vi "Configure Analog Out.vi"(0 "VISA resource name":refnum<visa-resource-name>, 1 "High Value (0.0000)":dbl min=-100000.0 max=100000.0 step=0.0001 format="%.4f", 2 "Low Value (0.0000)":dbl min=-100000.0 max=100000.0 step=0.0001 format="%.4f", 5 "Analog Out Mode (0: Off)":u16(ring) items=["Off", "Input", "Manual", "Loop 2"], 7 "Input (0: A)":u16(ring) items=["A", "B"], 9 "Source (0: Kelvin)":u16(ring) items=["Kelvin", "Celsius", "Sensor Units", "Linear Data"], 11 "error in (no error)":errorcluster, 12 "Bipolar Mode (F: OFF)":bool, 13 "Manual Value (0.000 %)":dbl min=-100.0 max=100.0 step=0.001 format="%.3f") -> (4 "VISA resource name out":refnum<visa-resource-name>, 15 "error out":errorcluster)   [LabVIEW 2013, in "Lake Shore Cryotronics 331.lvlib"]
doc: "This VI configures the 331 analog output. The analog output may be configured to send a voltage proportional to temperature to a strip chart recorder or data acquisition system The output can also be manually controlled as a voltage source for any other application or used as the countrol output for Loop 2."
uses:
  Lake Shore Cryotronics 331.lvlib
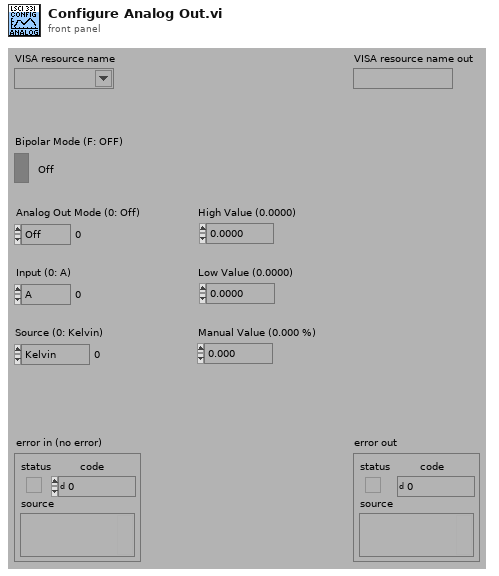
[diagram p1: front panel]
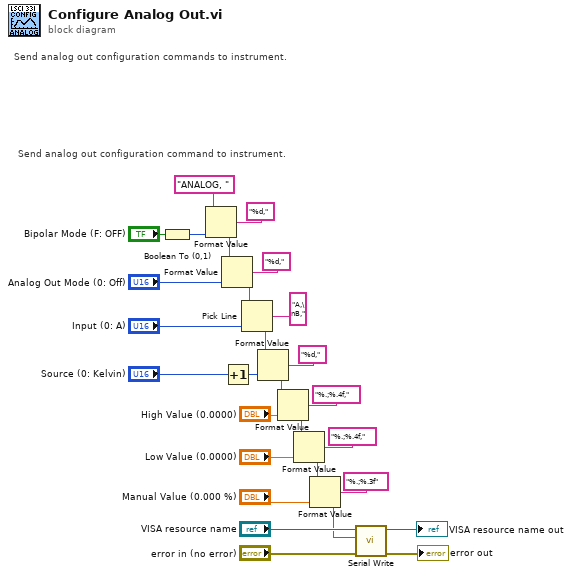
[diagram p0: block diagram]
diagram:
  # "Send analog out configuration command to instrument."
  # "Send analog out configuration commands to instrument."
  n1 = Boolean To (0,1)(Boolean="Bipolar Mode (F: OFF)") -> (0, 1=w21:i16)
  n2 = Format Value(string ("")="ANALOG, ", format string="%d,", value (0)=w21) -> (output string=w18:string)
  n3 = Format Value(string ("")=w18, format string="%d,", value (0)="Analog Out Mode (0: Off)") -> (output string=w15:string)
  n4 = Increment(x="Source (0: Kelvin)") -> (x+1=w11:u16)
  n5 = Pick Line(string ("")=w15, multi-line string="A,\nB,", line index="Input (0: A)") -> (output string=w12:string)
  n6 = Format Value(string ("")=w12, format string="%d,", value (0)=w11) -> (output string=w7:string)
  n7 = Format Value(string ("")=w7, format string="%.;%.4f,", value (0)="High Value (0.0000)") -> (output string=w6:string)
  n8 = Format Value(string ("")=w6, format string="%.;%.4f,", value (0)="Low Value (0.0000)") -> (output string=w5:string)
  n9 = Format Value(string ("")=w5, format string="%.;%.3f", value (0)="Manual Value (0.000 %)") -> (output string=w1:string)
  n10 = call "Serial Write.vi"("error in (no error)"="error in (no error)", "Write Buffer (\"\")"=w1, "VISA resource name"="VISA resource name") -> ("error out"=→"error out":errorcluster, "VISA resource name out"=→"VISA resource name out":refnum<visa-resource-name>)  [unwired: 6 in, 1 out]
